vi "Install or Uninstall Components 1.0.vi"(4 "Version Selection (Highest)":u32[](array[ring]) items=["Highest", "Exactly"], 6 "Auto-select Dependencies (T)":bool=TRUE, 7 "Restart Automatically (T)":bool=TRUE, 8 "error in (no error)":errorcluster, 9 "Software IDs to Uninstall":string[](array[string]), 10 "Software Components to Install":T2[](array[typedef]), 11 "Session in":refnum<k21>) -> (0 "error out":errorcluster, 1 "Broken Dependencies":T1[](array[typedef]), 3 "Session out":refnum<k21>)   [LabVIEW 2017, in "nisyscfg.lvlib"]
uses:
  <vilib>/nisyscfg/nisyscfg.lvlib
  <vilib>/nisyscfg/Software.ctl
  <vilib>/nisyscfg/Broken Dependency.ctl
  <vilib>/nisyscfg/Software 1.2.ctl
  <vilib>/nisyscfg/Component Type.ctl
  <vilib>/nisyscfg/Install or Uninstall Components.vi
panel:
  # "This cluster is deprecated.\nUse Broken Dependency 1.2.ctl."
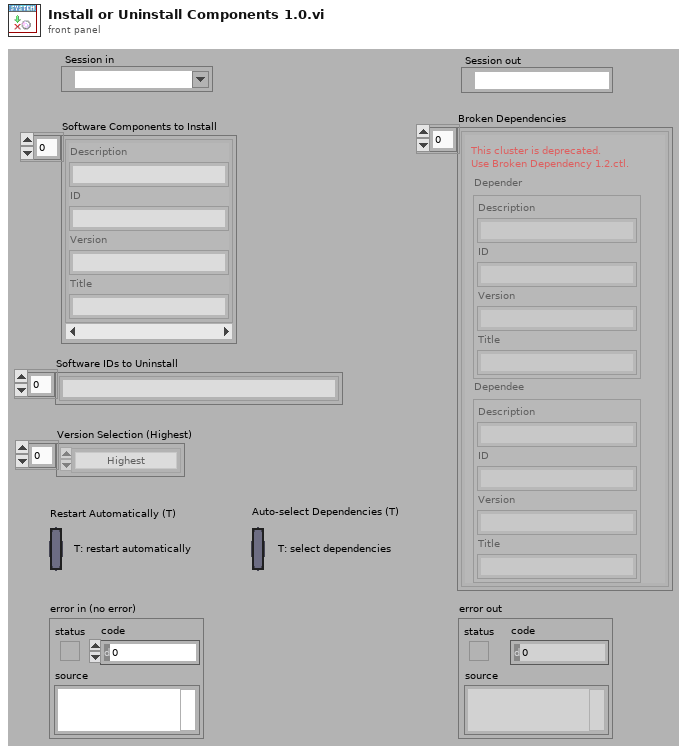
[diagram p1: front panel]
types:
  T1 = typedef "nisyscfg.lvlib/Broken Dependency.ctl" = cluster{"Depender":T2, "Dependee":T2}
  T2 = typedef "nisyscfg.lvlib/Software.ctl" = cluster{"Description":string, "ID":string, "Version":string, "Title":string}
  T3 = typedef "nisyscfg.lvlib/Software 1.2.ctl" = cluster{"title":string, "description":string, "ID":string, "version":string, "component type":T4}
  T4 = typedef "nisyscfg.lvlib/Component Type.ctl" = u32
  T5 = typedef "nisyscfg.lvlib/Broken Dependency 1.2.ctl" = cluster{"depender":T3, "dependee":T3}
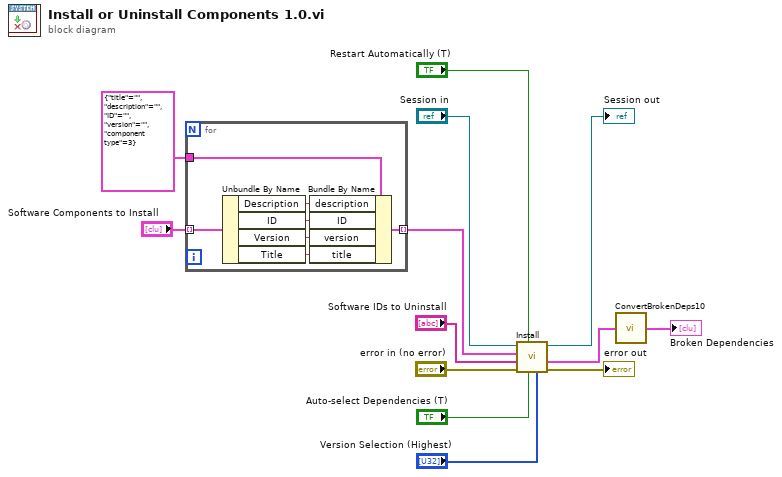
[diagram p0: block diagram]
diagram:
  n1 = for {
    tunnel: "Software Components to Install" -> [w20] mode=indexing
    tunnel: T3 {"title"="", "description"="", "ID"="", "version"="", "component type"=3} ("software") -> [w19]
    tunnel: [w14] -> w1 mode=indexing
    n2 = Unbundle By Name(w20) -> ("Description"=w18:string, "ID"=w17:string, "Version"=w16:string, "Title"=w15:string)
    n3 = Bundle By Name(cluster=w19, "description"=w18, "ID"=w17, "version"=w16, "title"=w15) -> (w14:T3)
  }
  n4 = call-poly <vilib>:"Install.vi"("Version Selection (Highest)"="Version Selection (Highest)", "Auto-select Dependencies (T)"="Auto-select Dependencies (T)", "Restart Automatically (T)"="Restart Automatically (T)", "error in (no error)"="error in (no error)", "Software IDs to Uninstall"="Software IDs to Uninstall", "Software Components to Install"=w1, "Session in"="Session in") -> ("error out"=→"error out":errorcluster, "Broken Dependencies"=w8:T5[], "Session out"=→"Session out":refnum<k21>)  [unwired: 2 in]
  n5 = call <vilib>:"ConvertBrokenDeps10.vi"("dependencies 1.2"=w8) -> ("dependencies 1.0"=→"Broken Dependencies":T1[])
